vi "Contains.vi"(8 "error in (no error)":errorcluster, 10 "Key":string, 11 "Array In":refnum<class "Array.lvclass">) -> (0 "error out":errorcluster, 1 "Key Exists?":bool, 3 "Array Out":refnum<class "Array.lvclass">)   [LabVIEW 2013, in "LapDog.Collections.v_.Maps.Implementations.lvlib" / "Array.lvclass"]
doc: "Returns a boolean True if the key exists in the map."
uses:
  Array.lvclass
  Array.lvclass/Array.ctl
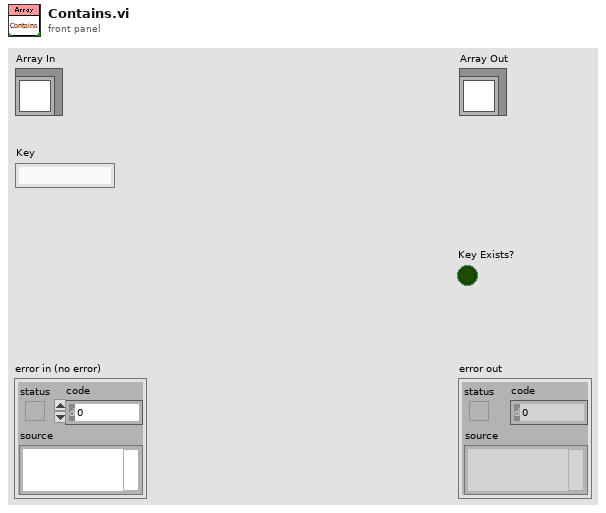
[diagram p1: front panel]
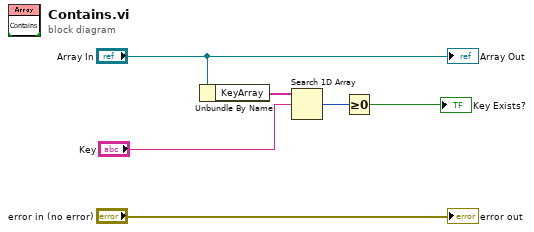
[diagram p0: block diagram]
diagram:
  n1 = Unbundle By Name("Array In") -> ("KeyArray"=w4:string[])
  n2 = Search 1D Array(1D array=w4, element="Key") -> (index of element=w2:i32)  [unwired: 1 in]
  n3 = Greater Or Equal To 0?(x=w2) -> (x >= 0?=→"Key Exists?":bool)
  "error out" <- "error in (no error)"
  "Array Out" <- "Array In"
